vi "Moisture_Init.vi"(0 "Physical Channel(s)":tag="Dev1/ao0", 11 "Error In":errorcluster) -> (4 "task out":refnum<k21>, 15 "Error Out":errorcluster)   [LabVIEW 2014]
uses:
  <vilib>/DAQmx/create/channels.llb/DAQmx Create Channel (AO-Voltage-Basic).vi
  <vilib>/DAQmx/configure/timing.llb/DAQmx Timing (Sample Clock).vi
  <resource>/objmgr/daqmx.rc
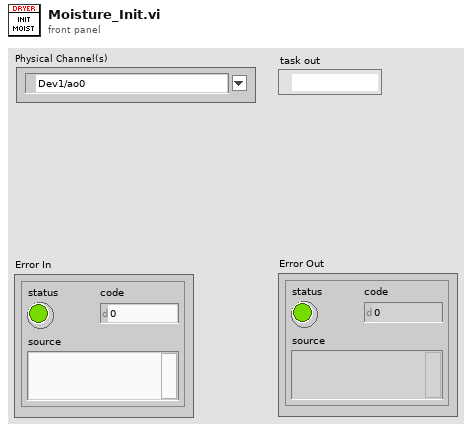
[diagram p1: front panel]
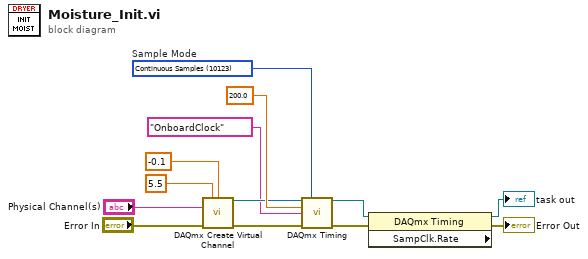
[diagram p0: block diagram]
diagram:
  w7 = 10123 items=["Finite Samples"=10178, "Continuous Samples"=10123, "Hardware Timed Single Point"=12522]  # Sample Mode
  n1 = call-poly <vilib>:"DAQmx Create Virtual Channel.vi"("maximum value"=5.5 ("Max Voltage"), "minimum value"=-0.1 ("Min Voltage"), "physical channels"="Physical Channel(s)", "error in"="Error In") -> ("task out"=w9:refnum<k21>, "error out"=w8:errorcluster)  [unwired: 10 in]
  n2 = call-poly <vilib>:"DAQmx Timing.vi"("task/channels in"=w9, "sample mode"=w7, "rate"=200.0 ("Sample Rate"), "source"=tag "OnboardClock", "error in"=w8) -> ("task out"=w5:refnum<k21>, "error out"=w6:errorcluster)  [unwired: 9 in]
  n3 = property class="DAQmx Timing" props=["SampClk.Rate"](reference=w5, error in=w6) -> (reference out=→"task out":refnum<k21>, error out=→"Error Out":errorcluster)  [unwired: 1 out]
